vi "USB2SPI.vi"() -> ()   [LabVIEW 2014]
uses:
  D:/ExpApp/AD5372/usb2uis.dll
panel:
  out "Version 2":string
  in  "Connect":bool
  in  "Exit":bool
  in  "Device No.":u8=255 format="%x"
  out "Serial No.":string
  in  "Select":u16(ring) items=["DLL", "SYS", "MCU"]
  in  "GetVersion":bool
  out "Version":string
  in  "read data":string="\u0000"
  in  "Write data":string="\u0000"
  in  "Write Command":string="\u0000"
  in  "SPIWrite":bool
  in  "Read Command":string="\u0000"
  in  "Length":u8=16
  in  "Mode":u16(ring) items=["Mode0(00)", "Mode1(01)", "Mode2(10)", "Mode3(11)"]
  in  "Frequency":u16(ring)=4 items=["200KHz", "400KHz", "600KHz", "800KHz", "1MHz", "2MHz", "4MHz", "6MHz", "12MHz"]
  in  "SetSPI":bool
  in  "SPIRead":bool
  # "USB2SPI Demo"
  # "Device Info"
  # "SPI Configuration"
  # "Version Read"
  # "SPI Read"
  # "SPI Write"
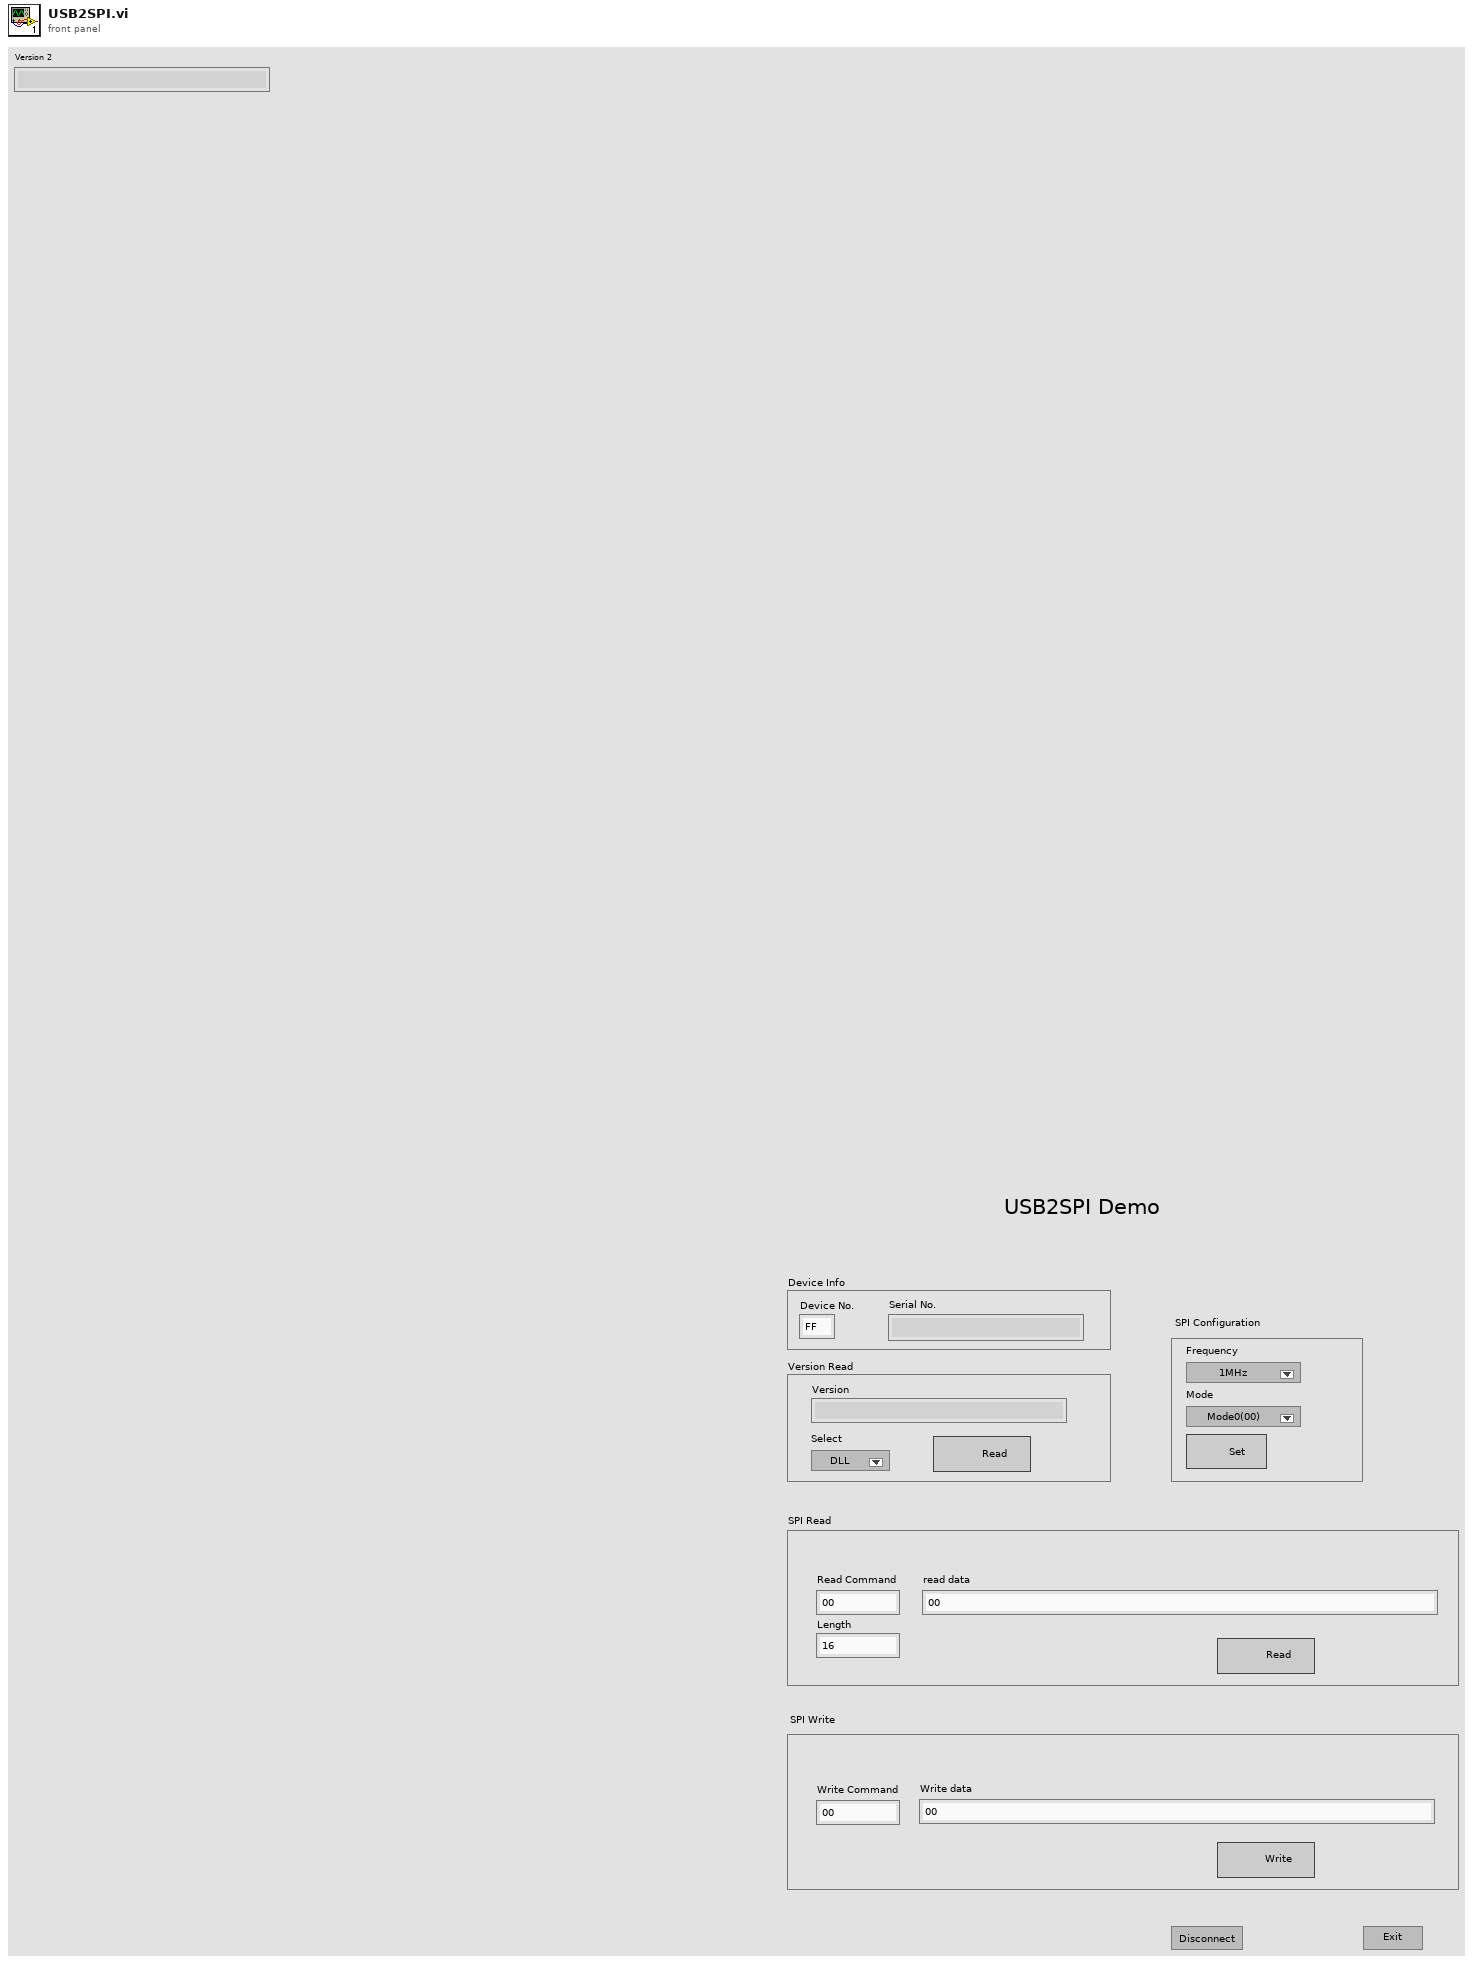
[diagram p1: front panel]
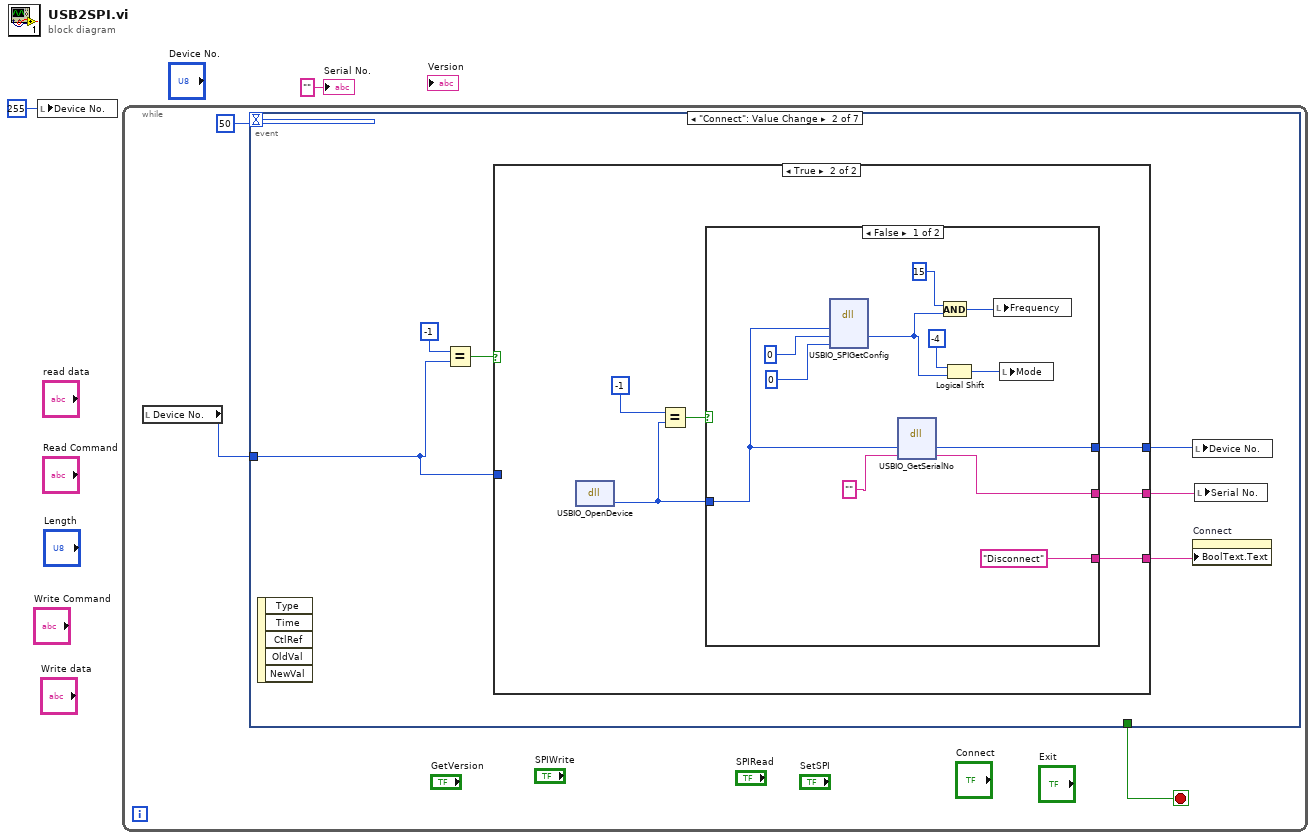
[diagram p0: block diagram]
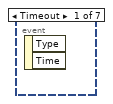
[diagram p2: hidden frame]
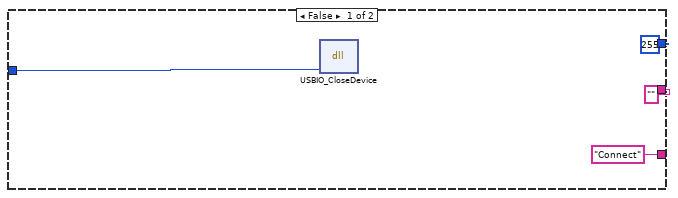
[diagram p3: hidden frame]
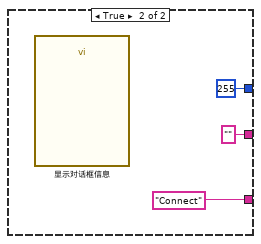
[diagram p4: hidden frame]
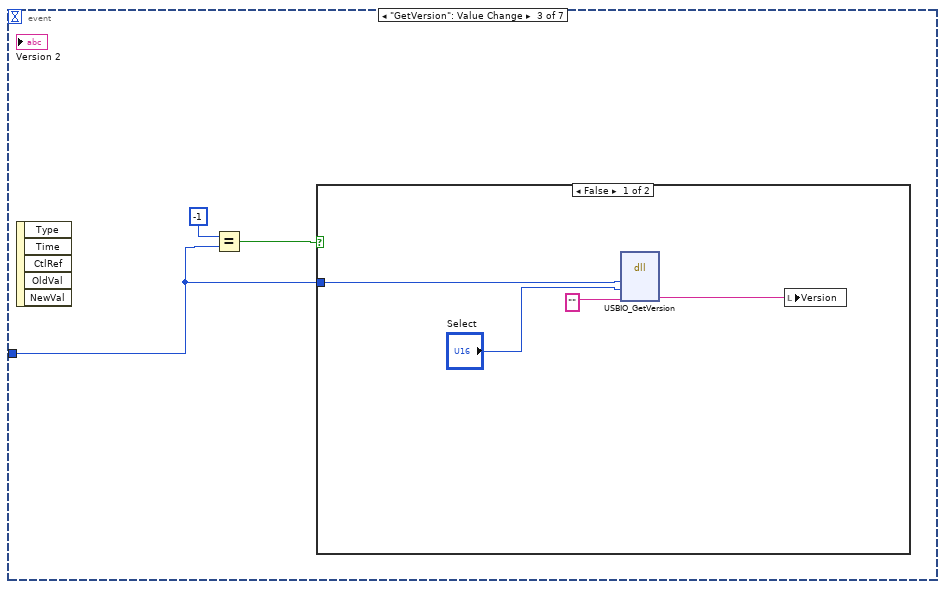
[diagram p5: hidden frame]
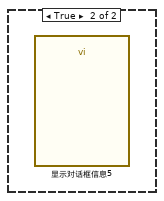
[diagram p6: hidden frame]
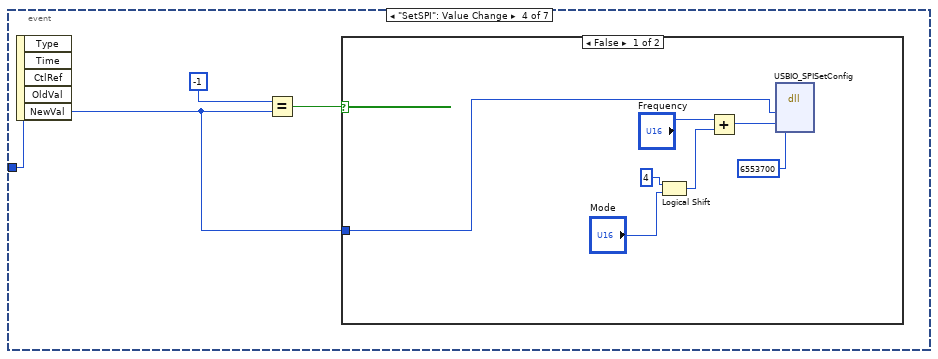
[diagram p7: hidden frame]
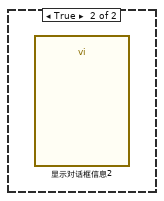
[diagram p8: hidden frame]
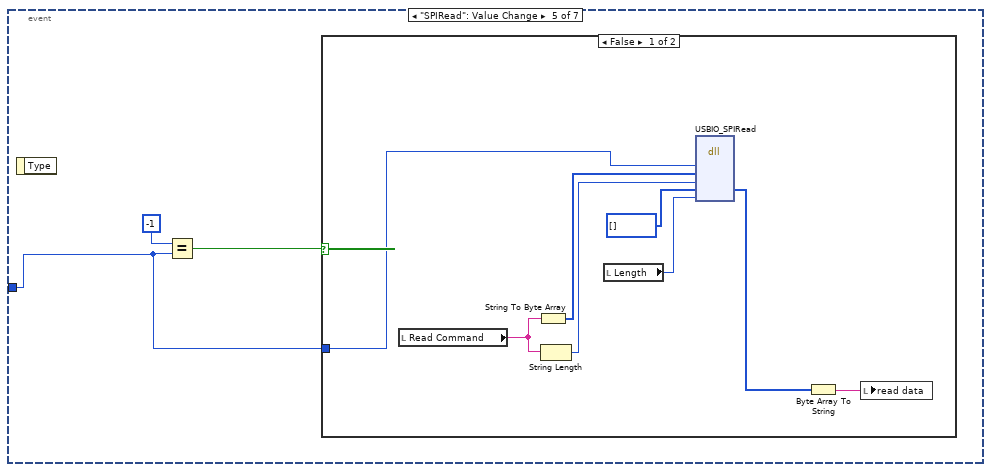
[diagram p9: hidden frame]
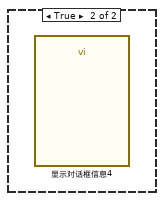
[diagram p10: hidden frame]
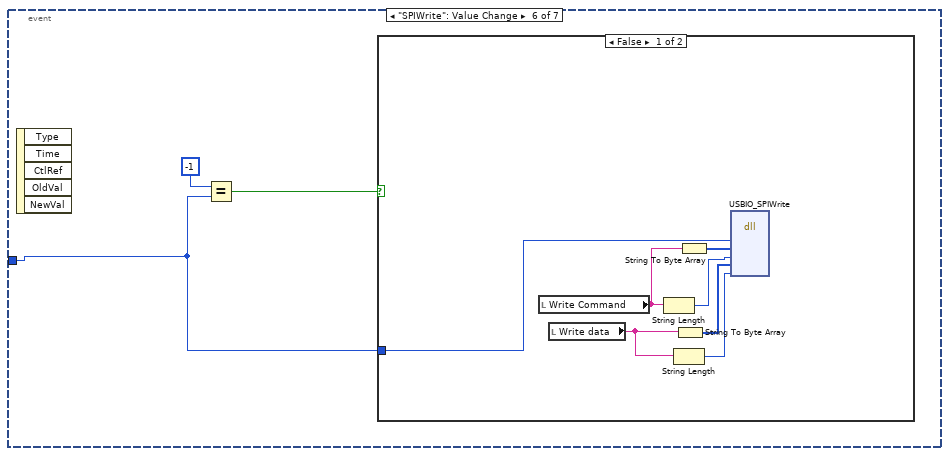
[diagram p11: hidden frame]
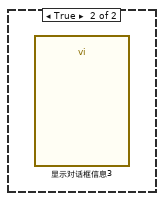
[diagram p12: hidden frame]
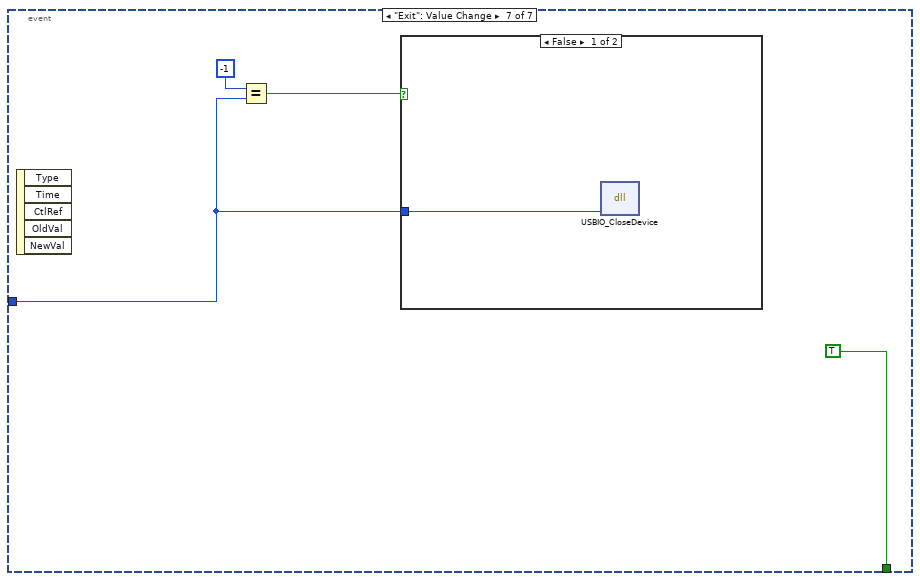
[diagram p13: hidden frame]
diagram:
  n1 = local write "Device No."(u8 255 ("Device No.")) -> ()
  n2 = while {
    stop <- w3 stop-if-true
    n3 = local read "Device No."() -> (w4:u8)
    n4 = event shown="[1] \"Connect\": Value Change" {
      selector: _ -> [_ _ _ _ _ _ _]
      dyn-events: _ -> [_ _ _ _ _ _ _]
      timeout: 50 -> [_ _ _ _ _ _ _]
      tunnel: w4 -> [_ w9 w37 w44 w54 w65 w76]
      tunnel: [_ _ _ _ _ _ TRUE] -> w3
      event Timeout {
        n5 = event-data() -> ()  [unwired: 1 in, 2 out]
      }
      event "Connect": Value Change {
        n6 = event-data() -> ()  [unwired: 1 in, 5 out]
        n7 = Equal?(x=i8 -1, y=w9) -> (x = y?=w10:bool)
        n8 = case shown="True" w10 {
          tunnel: [u8 255 ("u8DevIndex") w18] -> w8
          tunnel: ["" ("lpBuffer") w17] -> w7
          tunnel: w9 -> [w15 _]
          tunnel: ["Connect" ("Boolean Text.Text") w16] -> w6
          frame False {
            n9 = dll-call lib="D:/ExpApp/AD5372/usb2uis.dll" fn="USBIO_CloseDevice"("u8DevIndex"=w15) -> ()  [unwired: 5 in, 2 out]
          }
          frame True {
            n10 = dll-call lib="D:/ExpApp/AD5372/usb2uis.dll" fn="USBIO_OpenDevice"() -> ("返回类型"=w19:u8)  [unwired: 3 in, 2 out]
            n11 = Equal?(x=i8 -1, y=w19) -> (x = y?=w20:bool)
            n12 = case shown="False" w20 {
              tunnel: w19 -> [w29 _]
              tunnel: [w32 u8 255 ("u8DevIndex")] -> w18
              tunnel: [w31 "" ("lpBuffer")] -> w17
              tunnel: ["Disconnect" "Connect"] -> w16
              frame False {
                n13 = dll-call lib="D:/ExpApp/AD5372/usb2uis.dll" fn="USBIO_SPIGetConfig"("u8DevIndex"=w29, "pu8Rate"=u8 0, "pu32Timeout"=u32 0) -> ("pu8Rate"=w23:u8)  [unwired: 6 in, 2 out]
                n14 = dll-call lib="D:/ExpApp/AD5372/usb2uis.dll" fn="USBIO_GetSerialNo"("u8DevIndex"=w29, "lpBuffer"="") -> ("u8DevIndex"=w32:u8, "lpBuffer"=w31:string)  [unwired: 4 in, 2 out]
                n15 = And(x=u8 15, y=w23) -> (x .and. y?=w26:u8)
                n16 = Logical Shift(y=i16 -4, x=w23) -> (x << y=w24:u8)
                n17 = local write "Frequency"(w26) -> ()
                n18 = local write "Mode"(w24) -> ()
              }
              frame True {
                n19 = call "显示对话框信息"() -> ()  [unwired: 10 in, 2 out]
              }
            }
          }
        }
        n20 = local write "Device No."(w8) -> ()
        n21 = property on="Connect" class="Bool"("BoolText.Text"=w6) -> ()  [unwired: 2 in, 2 out]
        n22 = local write "Serial No."(w7) -> ()
      }
      event "GetVersion": Value Change {
        n23 = event-data() -> ()  [unwired: 1 in, 5 out]
        n24 = Equal?(x=i8 -1, y=w37) -> (x = y?=w38:bool)
        n25 = case shown="False" w38 {
          tunnel: w37 -> [w42 _]
          frame False {
            n26 = dll-call lib="D:/ExpApp/AD5372/usb2uis.dll" fn="USBIO_GetVersion"("u8DevIndex"=w42, "Type"="Select", "lpBuffer"="") -> ("lpBuffer"=w40:string)  [unwired: 6 in, 2 out]
            n27 = local write "Version"(w40) -> ()
          }
          frame True {
            n28 = call "显示对话框信息5"() -> ()  [unwired: 10 in, 2 out]
          }
        }
      }
      event "SetSPI": Value Change {
        n29 = event-data() -> ()  [unwired: 1 in, 5 out]
        n30 = Equal?(x=i8 -1, y=w44) -> (x = y?=w45:bool)
        n31 = case shown="False" w45 {
          tunnel: w44 -> [w47 _]
          frame False {
            n32 = Logical Shift(y=i8 4, x="Mode") -> (x << y=w51:u16)
            n33 = Add(x="Frequency", y=w51) -> (x+y=w52:u16)
            n34 = dll-call lib="D:/ExpApp/AD5372/usb2uis.dll" fn="USBIO_SPISetConfig"("u8DevIndex"=w47, "u8Value"=w52, "u32Timeout"=6553700) -> ()  [unwired: 7 in, 2 out]
          }
          frame True {
            n35 = call "显示对话框信息2"() -> ()  [unwired: 10 in, 2 out]
          }
        }
      }
      event "SPIRead": Value Change {
        n36 = event-data() -> ()  [unwired: 1 in, 1 out]
        n37 = Equal?(x=i8 -1, y=w54) -> (x = y?=w55:bool)
        n38 = case shown="False" w55 {
          tunnel: w54 -> [w60 _]
          frame False {
            n39 = local read "Read Command"() -> (w64:string)
            n40 = String To Byte Array(string=w64) -> (unsigned byte array=w59:u8[])
            n41 = String Length(string=w64) -> (length=w58:i32)
            n42 = local read "Length"() -> (w61:u8)
            n43 = dll-call lib="D:/ExpApp/AD5372/usb2uis.dll" fn="USBIO_SPIRead"("u8DevIndex"=w60, "lpParaBuffer"=w59, "ParaSize"=w58, "lpReadBuffer"=u8[] [], "wReadSize"=w61) -> ("lpReadBuffer"=w57:u8[])  [unwired: 8 in, 2 out]
            n44 = Byte Array To String(unsigned byte array=w57) -> (string=w63:string)
            n45 = local write "read data"(w63) -> ()
          }
          frame True {
            n46 = call "显示对话框信息4"() -> ()  [unwired: 10 in, 2 out]
          }
        }
      }
      event "SPIWrite": Value Change {
        n47 = event-data() -> ()  [unwired: 1 in, 5 out]
        n48 = Equal?(x=i8 -1, y=w65) -> (x = y?=w66:bool)
        n49 = case shown="False" w66 {
          tunnel: w65 -> [w74 _]
          frame False {
            n50 = local read "Write Command"() -> (w71:string)
            n51 = local read "Write data"() -> (w70:string)
            n52 = String Length(string=w71) -> (length=w72:i32)
            n53 = String Length(string=w70) -> (length=w69:i32)
            n54 = String To Byte Array(string=w70) -> (unsigned byte array=w68:u8[])
            n55 = String To Byte Array(string=w71) -> (unsigned byte array=w73:u8[])
            n56 = dll-call lib="D:/ExpApp/AD5372/usb2uis.dll" fn="USBIO_SPIWrite"("u8DevIndex"=w74, "lpParaBuffer"=w73, "ParaSize"=w72, "lpWriteBuffer"=w68, "wWriteSize"=w69) -> ()  [unwired: 9 in, 2 out]
          }
          frame True {
            n57 = call "显示对话框信息3"() -> ()  [unwired: 10 in, 2 out]
          }
        }
      }
      event "Exit": Value Change {
        n58 = event-data() -> ()  [unwired: 1 in, 5 out]
        n59 = Equal?(x=i8 -1, y=w76) -> (x = y?=w77:bool)
        n60 = case shown="False" w77 {
          tunnel: w76 -> [w79 _]
          frame False {
            n61 = dll-call lib="D:/ExpApp/AD5372/usb2uis.dll" fn="USBIO_CloseDevice"("u8DevIndex"=w79) -> ()  [unwired: 5 in, 2 out]
          }
          frame True {
          }
        }
      }
    }
  }
  "Serial No." <- "" ("Serial No.")
